vi "From Float Tree Data.vi"(11 "Tree Data":refnum<class "Tree Data.lvclass">) -> (2 "Float":dbl)   [LabVIEW 2016, in "Float.lvclass"]
uses:
  Float.lvclass
  Tree Data/Tree Data.lvclass
  Float.lvclass/Float.ctl
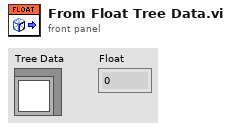
[diagram p1: front panel]
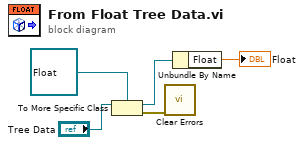
[diagram p0: block diagram]
diagram:
  n1 = To More Specific Class(target class=refnum<class "Float.lvclass"> refnum ("Float.lvclass"), reference="Tree Data") -> (specific class reference=w4:refnum<class "Float.lvclass">, error out=w3:errorcluster)  [unwired: 1 in]
  n2 = call <vilib>:"Clear Errors.vi"("error in (no error)"=w3) -> ()  [unwired: 5 in, 2 out]
  n3 = Unbundle By Name(w4) -> ("Float"=→"Float":dbl)
